vi "Get_Tree_Item.vi"(8 "error in (no error)":errorcluster, 11 "IB_TreeItem in":refnum<class "IB_Tree_Item.lvclass">) -> (0 "error out":errorcluster, 2 "data":T1, 3 "IB_TreeItem out":refnum<class "IB_Tree_Item.lvclass">)   [LabVIEW 2020, in "IB_Tree_Item.lvclass"]
uses:
  <vilib>/AppBuilder/IB_Classes/Tree_Item/IB_Tree_Item.lvclass
  <vilib>/AppBuilder/IB_Classes/Tree_Item/IB_Tree_Item.lvclass/IB_Tree_Item.ctl
  <vilib>/AppBuilder/IB_Classes/Tree_Item/IB_Tree_Item.ctl
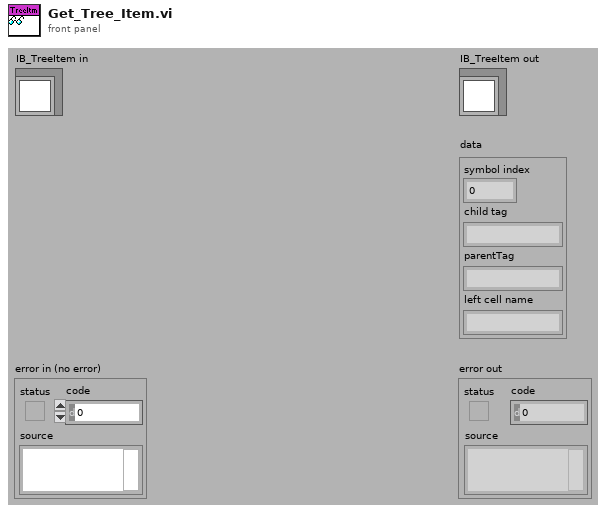
[diagram p1: front panel]
types:
  T1 = typedef "IB_Tree_Item.ctl" = cluster{"symbol index":i32, "child tag":string, "parentTag":string, "left cell name":string}
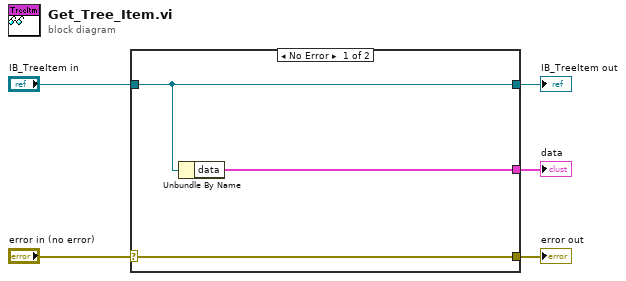
[diagram p0: block diagram]
diagram:
  n1 = case shown="No Error" "error in (no error)" {
    selector: "error in (no error)" -> [w8 w9]
    tunnel: [w8 w9] -> w4
    tunnel: [w7 w10] -> w2
    tunnel: "IB_TreeItem in" -> [w7 w10]
    tunnel: [w6 _] -> w1
    frame No Error {
      n2 = Unbundle By Name(w7) -> ("data"=w6:T1)
    }
    frame Error {
    }
  }
  "error out" <- w4
  "IB_TreeItem out" <- w2
  "data" <- w1
